vi "Weather Parse Test.vi"() -> ()   [LabVIEW 2020, in "CDM-Config.lvlib"] (continued)
008043\",\n                        \"008027\",\n                        \"008119\",\n                        \"008041\",\n                        \"008101\"\n                    ],\n                    \"UGC\": [\n                        \"COZ062\",\n                        \"COZ077\",\n                        \"COZ083\",\n                        \"COZ085\",\n                        \"COZ086\"\n                    ]\n                },\n                \"affectedZones\": [\n                    \"https://api.weather.gov/zones/forecast/COZ062\",\n                    \"https://api.weather.gov/zones/forecast/COZ077\",\n                    \"https://api.weather.gov/zones/forecast/COZ083\",\n                    \"https://api.weather.gov/zones/forecast/COZ085\",\n                    \"https://api.weather.gov/zones/forecast/COZ086\"\n                ],\n                \"references\": [\n                    {\n                        \"@id\": \"https://api.weather.gov/alerts/urn:oid:2.49.0.1.840.0.f1520a771888f2286c7e9f041b0899cca2ffbe10.006.1\",\n                        \"identifier\": \"urn:oid:2.49.0.1.840.0.f1520a771888f2286c7e9f041b0899cca2ffbe10.006.1\",\n                        \"sender\": \"w-nws.webmaster@noaa.gov\",\n                        \"sent\": \"2025-12-03T00:40:00-07:00\"\n                    },\n                    {\n                        \"@id\": \"https://api.weather.gov/alerts/urn:oid:2.49.0.1.840.0.3e97ab4a6a3c23a3a20405d82b018ef9927db31d.006.1\",\n                        \"identifier\": \"urn:oid:2.49.0.1.840.0.3e97ab4a6a3c23a3a20405d82b018ef9927db31d.006.1\",\n                        \"sender\": \"w-nws.webmaster@noaa.gov\",\n                        \"sent\": \"2025-12-03T00:46:00-07:00\"\n                    },\n                    {\n                        \"@id\": \"https://api.weather.gov/alerts/urn:oid:2.49.0.1.840.0.b7b2384d0cd65fff536137c85933eace889e9254.006.1\",\n                        \"identifier\": \"urn:oid:2.49.0.1.840.0.b7b2384d0cd65fff536137c85933eace889e9254.006.1\",\n                        \"sender\": \"w-nws.webmaster@noaa.gov\",\n                        \"sent\": \"2025-12-03T00:53:00-07:00\"\n                    },\n                    {\n                        \"@id\": \"https://api.weather.gov/alerts/urn:oid:2.49.0.1.840.0.5bb2b589973a618ffa88ed552c21d1806fce1897.006.1\",\n                        \"identifier\": \"urn:oid:2.49.0.1.840.0.5bb2b589973a618ffa88ed552c21d1806fce1897.006.1\",\n                        \"sender\": \"w-nws.webmaster@noaa.gov\",\n                        \"sent\": \"2025-12-03T02:10:00-07:00\"\n                    }\n                ],\n                \"sent\": \"2025-12-03T08:17:00-07:00\",\n                \"effective\": \"2025-12-03T08:17:00-07:00\",\n                \"onset\": \"2025-12-03T08:17:00-07:00\",\n                \"expires\": \"2025-12-03T16:30:00-07:00\",\n                \"ends\": \"2025-12-03T20:00:00-07:00\",\n                \"status\": \"Actual\",\n                \"messageType\": \"Update\",\n                \"category\": \"Met\",\n                \"severity\": \"Moderate\",\n                \"certainty\": \"Likely\",\n                \"urgency\": \"Expected\",\n                \"event\": \"Winter Weather Advisory\",\n                \"sender\": \"w-nws.webmaster@noaa.gov\",\n                \"senderName\": \"NWS Pueblo CO\",\n                \"headline\": \"Winter Weather Advisory issued December 3 at 8:17AM MST until December 3 at 8:00PM MST by NWS Pueblo CO\",\n                \"description\": \"* WHAT...Snow expected. Total snow accumulations between 2 and 8\\ninches. The heaviest snow will fall this morning into the\\nafternoon time period.\\n\\n* WHERE...Southern El Paso, Pueblo, Central Chaffee County Below\\n9000 Feet, Western/Central Fremont County Below 8500 Feet, and\\nCanon City Vicinity/Eastern Fremont County.\\n\\n* WHEN...Until 8 PM MST this evening.\\n\\n* IMPACTS...Roads, and especially bridges and overpasses, will\\nlikely become slick and hazardous. Travel could be very difficult.\\nThe hazardous conditions could impact the Wednesday evening\\ncommute.\",\n                \"instruction\": \"Slow down and use caution while traveling. The latest road\\nconditions for the state you are calling from can be obtained by\\ncalling 5 1 1.\\n\\nBe prepared for slippery roads. Slow down and use caution while\\ndriving. If you are going outside, watch your first few steps taken\\non stairs, sidewalks, and driveways. These surfaces could be icy and\\nslippery, increasing your risk of a fall and injury.\",\n                \"response\": \"Execute\",\n                \"parameters\": {\n                    \"AWIPSidentifier\": [\n                        \"WSWPUB\"\n                    ],\n                    \"WMOidentifier\": [\n                        \"WWUS45 KPUB 031517\"\n                    ],\n                    \"NWSheadline\": [\n                        \"WINTER WEATHER ADVISORY REMAINS IN EFFECT UNTIL 8 PM MST THIS EVENING\"\n                    ],\n                    \"BLOCKCHANNEL\": [\n                        \"EAS\",\n                        \"NWEM\",\n                        \"CMAS\"\n                    ],\n                    \"VTEC\": [\n                        \"/O.CON.KPUB.WW.Y.0026.000000T0000Z-251204T0300Z/\"\n                    ],\n                    \"eventEndingTime\": [\n                        \"2025-12-03T20:00:00-07:00\"\n                    ],\n                    \"expiredReferences\": [\n                        \"w-nws.webmaster@noaa.gov,urn:oid:2.49.0.1.840.0.1683fac8dbbcced155b8c3ee102b504a61d03b48.005.1,2025-12-02T21:22:00-07:00 w-nws.webmaster@noaa.gov,urn:oid:2.49.0.1.840.0.3af7c19979dcb0fd957b60f169e1bc971c265b37.007.1,2025-12-02T14:07:00-07:00 w-nws.webmaster@noaa.gov,urn:oid:2.49.0.1.840.0.3af7c19979dcb0fd957b60f169e1bc971c265b37.004.1,2025-12-02T14:07:00-07:00 w-nws.webmaster@noaa.gov,urn:oid:2.49.0.1.840.0.75fd3b8a9564f5fec4e84cc777455f52675d243c.003.1,2025-12-02T10:18:00-07:00 w-nws.webmaster@noaa.gov,urn:oid:2.49.0.1.840.0.db6c9ff9aeb621cf1cd0d104f439c64f55e7c3f7.003.1,2025-12-02T02:25:00-07:00\"\n                    ]\n                },\n                \"scope\": \"Public\",\n                \"code\": \"IPAWSv1.0\",\n                \"language\": \"en-US\",\n                \"web\": \"http://www.weather.gov\",\n                \"eventCode\": {\n                    \"SAME\": [\n                        \"NWS\"\n                    ],\n                    \"NationalWeatherService\": [\n                        \"WWY\"\n                    ]\n                }\n            }\n        },\n        {\n            \"id\": \"https://api.weather.gov/alerts/urn:oid:2.49.0.1.840.0.296069c17a90f6e5215450afb7029362483104e1.007.1\",\n            \"type\": \"Feature\",\n            \"geometry\": null,\n            \"properties\": {\n                \"@id\": \"https://api.weather.gov/alerts/urn:oid:2.49.0.1.840.0.296069c17a90f6e5215450afb7029362483104e1.007.1\",\n                \"@type\": \"wx:Alert\",\n                \"id\": \"urn:oid:2.49.0.1.840.0.296069c17a90f6e5215450afb7029362483104e1.007.1\",\n                \"areaDesc\": \"Northwestern Fremont County  Above 8500Ft\",\n                \"geocode\": {\n                    \"SAME\": [\n                        \"008043\"\n                    ],\n                    \"UGC\": [\n                        \"COZ076\"\n                    ]\n                },\n                \"affectedZones\": [\n                    \"https://api.weather.gov/zones/forecast/COZ076\"\n                ],\n                \"references\": [\n                    {\n                        \"@id\": \"https://api.weather.gov/alerts/urn:oid:2.49.0.1.840.0.f1520a771888f2286c7e9f041b0899cca2ffbe10.004.1\",\n                        \"identifier\": \"urn:oid:2.49.0.1.840.0.f1520a771888f2286c7e9f041b0899cca2ffbe10.004.1\",\n                        \"sender\": \"w-nws.webmaster@noaa.gov\",\n                        \"sent\": \"2025-12-03T00:40:00-07:00\"\n                    },\n                    {\n                        \"@id\": \"https://api.weather.gov/alerts/urn:oid:2.49.0.1.840.0.3e97ab4a6a3c23a3a20405d82b018ef9927db31d.004.1\",\n                        \"identifier\": \"urn:oid:2.49.0.1.840.0.3e97ab4a6a3c23a3a20405d82b018ef9927db31d.004.1\",\n                        \"sender\": \"w-nws.webmaster@noaa.gov\",\n                        \"sent\": \"2025-12-03T00:46:00-07:00\"\n                    },\n                    {\n                        \"@id\": \"https://api.weather.gov/alerts/urn:oid:2.49.0.1.840.0.b7b2384d0cd65fff536137c85933eace889e9254.004.1\",\n                        \"identifier\": \"urn:oid:2.49.0.1.840.0.b7b2384d0cd65fff536137c85933eace889e9254.004.1\",\n                        \"sender\": \"w-nws.webmaster@noaa.gov\",\n                        \"sent\": \"2025-12-03T00:53:00-07:00\"\n                    },\n                    {\n                        \"@id\": \"https://api.weather.gov/alerts/urn:oid:2.49.0.1.840.0.5bb2b589973a618ffa88ed552c21d1806fce1897.003.1\",\n                        \"identifier\": \"urn:oid:2.49.0.1.840.0.5bb2b589973a618ffa88ed552c21d1806fce1897.003.1\",\n                        \"sender\": \"w-nws.webmaster@noaa.gov\",\n                        \"sent\": \"2025-12-03T02:10:00-07:00\"\n                    }\n                ],\n                \"sent\": \"2025-12-03T08:17:00-07:00\",\n                \"effective\": \"2025-12-03T08:17:00-07:00\",\n                \"onset\": \"2025-12-03T08:17:00-07:00\",\n                \"expires\": \"2025-12-03T16:30:00-07:00\",\n                \"ends\": \"2025-12-03T20:00:00-07:00\",\n                \"status\": \"Actual\",\n                \"messageType\": \"Update\",\n                \"category\": \"Met\",\n                \"severity\": \"Moderate\",\n                \"certainty\": \"Likely\",\n                \"urgency\": \"Expected\",\n                \"event\": \"Winter Weather Advisory\",\n                \"sender\": \"w-nws.webmaster@noaa.gov\",\n                \"senderName\": \"NWS Pueblo CO\",\n                \"headline\": \"Winter Weather Advisory issued December 3 at 8:17AM MST until December 3 at 8:00PM MST by NWS Pueblo CO\",\n                \"description\": \"* WHAT...Snow. Additional snow accumulations between 5 to 10 inches.\\n\\n* WHERE...Northwestern Fremont County Above 8500 Feet.\\n\\n* WHEN...Until 8 PM MST this evening.\\n\\n* IMPACTS...Travel could be very difficult. The hazardous conditions\\ncould impact the Wednesday evening commute.\",\n                \"instruction\": \"Slow down and use caution while traveling. The latest road\\nconditions for the state you are calling from can be obtained by\\ncalling 5 1 1.\",\n                \"response\": \"Execute\",\n                \"parameters\": {\n                    \"AWIPSidentifier\": [\n                        \"WSWPUB\"\n                    ],\n                    \"WMOidentifier\": [\n                        \"WWUS45 KPUB 031517\"\n                    ],\n                    \"NWSheadline\": [\n                        \"WINTER WEATHER ADVISORY REMAINS IN EFFECT UNTIL 8 PM MST THIS EVENING\"\n                    ],\n                    \"BLOCKCHANNEL\": [\n                        \"EAS\",\n                        \"NWEM\",\n                        \"CMAS\"\n                    ],\n                    \"VTEC\": [\n                        \"/O.CON.KPUB.WW.Y.0026.000000T0000Z-251204T0300Z/\"\n                    ],\n                    \"eventEndingTime\": [\n                        \"2025-12-03T20:00:00-07:00\"\n                    ],\n                    \"expiredReferences\": [\n                        \"w-nws.webmaster@noaa.gov,urn:oid:2.49.0.1.840.0.1683fac8dbbcced155b8c3ee102b504a61d03b48.003.1,2025-12-02T21:22:00-07:00 w-nws.webmaster@noaa.gov,urn:oid:2.49.0.1.840.0.3af7c19979dcb0fd957b60f169e1bc971c265b37.003.1,2025-12-02T14:07:00-07:00\"\n                    ]\n                },\n                \"scope\": \"Public\",\n                \"code\": \"IPAWSv1.0\",\n                \"language\": \"en-US\",\n                \"web\": \"http://www.weather.gov\",\n                \"eventCode\": {\n                    \"SAME\": [\n                        \"NWS\"\n                    ],\n                    \"NationalWeatherService\": [\n                        \"WWY\"\n                    ]\n                }\n            }\n        },\n        {\n            \"id\": \"https://api.weather.gov/alerts/urn:oid:2.49.0.1.840.0.2ecab18b7c46d70605970fa14b41f00f24fa37fd.001.1\",\n            \"type\": \"Feature\",\n            \"geometry\": null,\n            \"properties\": {\n                \"@id\": \"https://api.weather.gov/alerts/urn:oid:2.49.0.1.840.0.2ecab18b7c46d70605970fa14b41f00f24fa37fd.001.1\",\n                \"@type\": \"wx:Alert\",\n                \"id\": \"urn:oid:2.49.0.1.840.0.2ecab18b7c46d70605970fa14b41f00f24fa37fd.001.1\",\n                \"areaDesc\": \"Coastal Gulf\",\n                \"geocode\": {\n                    \"SAME\": [\n                        \"012045\"\n                    ],\n                    \"UGC\": [\n                        \"FLZ114\"\n                    ]\n                },\n                \"affectedZones\": [\n                    \"https://api.weather.gov/zones/forecast/FLZ114\"\n                ],\n                \"references\": [],\n                \"sent\": \"2025-12-03T09:59:00-05:00\",\n                \"effective\": \"2025-12-03T09:59:00-05:00\",\n                \"onset\": \"2025-12-03T09:59:00-05:00\",\n                \"expires\": \"2025-12-03T21:00:00-05:00\",\n                \"ends\": \"2025-12-03T21:00:00-05:00\",\n                \"status\": \"Actual\",\n                \"messageType\": \"Alert\",\n                \"category\": \"Met\",\n                \"severity\": \"Moderate\",\n                \"certainty\": \"Likely\",\n                \"urgency\": \"Expected\",\n                \"event\": \"Rip Current Statement\",\n                \"sender\": \"w-nws.webmaster@noaa.gov\",\n                \"senderName\": \"NWS Tallahassee FL\",\n                \"headline\": \"Rip Current Statement issued December 3 at 9:59AM EST until December 3 at 9:00PM EST by NWS Tallahassee FL\",\n                \"description\": \"* WHAT...Dangerous rip currents.\\n\\n* WHERE...Gulf County State Park Beaches.\\n\\n* WHEN...Until 9 PM EST /8 PM CST/ this evening.\\n\\n* IMPACTS...Rip currents can sweep even the best swimmers away\\nfrom shore into deeper water.\",\n                \"instruction\": \"Swim near a lifeguard. If caught in a rip current, relax and\\nfloat. Don't swim against the current. If able, swim in a\\ndirection following the shoreline. If unable to escape, face the\\nshore and call or wave for help.\",\n                \"response\": \"Avoid\",\n                \"parameters\": {\n                    \"AWIPSidentifier\": [\n                        \"CFWTAE\"\n                    ],\n                    \"WMOidentifier\": [\n                        \"WHUS42 KTAE 031459\"\n                    ],\n                    \"NWSheadline\": [\n                        \"HIGH RIP CURRENT RISK IN EFFECT UNTIL 9 PM EST /8 PM CST/ THIS EVENING\"\n                    ],\n                    \"BLOCKCHANNEL\": [\n                        \"EAS\",\n                        \"NWEM\",\n                        \"CMAS\"\n                    ],\n                    \"VTEC\": [\n                        \"/O.NEW.KTAE.RP.S.0089.251203T1459Z-251204T0200Z/\"\n                    ],\n                    \"eventEndingTime\": [\n                        \"2025-12-03T21:00:00-05:00\"\n                    ]\n                },\n                \"scope\": \"Public\",\n                \"code\": \"IPAWSv1.0\",\n                \"language\": \"en-US\",\n                \"web\": \"http://www.weather.gov\",\n                \"eventCode\": {\n                    \"SAME\": [\n                        \"NWS\"\n                    ],\n                    \"NationalWeatherService\": [\n                        \"RPS\"\n                    ]\n                }\n            }\n        },\n        {\n            \"id\": \"https://api.weather.gov/alerts/urn:oid:2.49.0.1.840.0.2ef41cb89e608f983559be19a65d260c36845a4b.001.2\",\n            \"type\": \"Feature\",\n            \"geometry\": null,\n            \"properties\": {\n                \"@id\": \"https://api.weather.gov/alerts/urn:oid:2.49.0.1.840.0.2ef41cb89e608f983559be19a65d260c36845a4b.001.2\",\n                \"@type\": \"wx:Alert\",\n                \"id\": \"urn:oid:2.49.0.1.840.0.2ef41cb89e608f983559be19a65d260c36845a4b.001.2\",\n                \"areaDesc\": \"Coastal Waters from Eastport, ME to Schoodic Point, ME out 25 NM; Coastal Waters from Schoodic Point, ME to Stonington, ME out 25 NM\",\n                \"geocode\": {\n                    \"SAME\": [\n                        \"073050\",\n                        \"073051\"\n                    ],\n                    \"UGC\": [\n                        \"ANZ050\",\n                        \"ANZ051\"\n                    ]\n                },\n                \"affectedZones\": [\n                    \"https://api.weather.gov/zones/forecast/ANZ050\",\n                    \"https://api.weather.gov/zones/forecast/ANZ051\"\n                ],\n                \"references\": [],\n                \"sent\": \"2025-12-03T09:58:00-05:00\",\n                \"effective\": \"2025-12-03T09:58:00-05:00\",\n                \"onset\": \"2025-12-04T15:00:00-05:00\",\n                \"expires\": \"2025-12-03T18:00:00-05:00\",\n                \"ends\": \"2025-12-05T07:00:00-05:00\",\n                \"status\": \"Actual\",\n                \"messageType\": \"Alert\",\n                \"category\": \"Met\",\n                \"severity\": \"Moderate\",\n                \"certainty\": \"Likely\",\n                \"urgency\": \"Expected\",\n                \"event\": \"Gale Warning\",\n                \"sender\": \"w-nws.webmaster@noaa.gov\",\n                \"senderName\": \"NWS Caribou ME\",\n                \"headline\": \"Gale Warning issued December 3 at 9:58AM EST until December 5 at 7:00AM EST by NWS Caribou ME\",\n                \"description\": \"* WHAT...Northwest winds 30 to 40 kt and seas 7 to 10 ft\\nexpected.\\n\\n* WHERE...Coastal Waters from Eastport, ME to Schoodic Point, ME\\nout 25 NM and Coastal Waters from Schoodic Point, ME to\\nStonington, ME out 25 NM.\\n\\n* WHEN...From 3 PM Thursday to 7 AM EST Friday.\\n\\n* IMPACTS...Strong winds will cause hazardous seas which could\\ncapsize or damage vessels and reduce visibility.\",\n                \"instruction\": \"Mariners should alter plans to avoid these hazardous conditions.\\nRemain in port, seek safe harbor, alter course, and/or secure the\\nvessel for hazardous conditions.\",\n                \"response\": \"Avoid\",\n                \"parameters\": {\n                    \"AWIPSidentifier\": [\n                        \"MWWCAR\"\n                    ],\n                    \"WMOidentifier\": [\n                        \"WHUS71 KCAR 031458\"\n                    ],\n                    \"NWSheadline\": [\n                        \"GALE WARNING WILL EXPIRE AT 10 AM EST THIS MORNING... ...GALE WARNING IN EFFECT FROM 3 PM THURSDAY TO 7 AM EST FRIDAY\"\n                    ],\n                    \"BLOCKCHANNEL\": [\n                        \"EAS\",\n                        \"NWEM\",\n                        \"CMAS\"\n                    ],\n                    \"VTEC\": [\n                        \"/O.NEW.KCAR.GL.W.0035.251204T2000Z-251205T1200Z/\"\n                    ],\n                    \"eventEndingTime\": [\n                        \"2025-12-05T07:00:00-05:00\"\n                    ]\n                },\n                \"scope\": \"Public\",\n                \"code\": \"IPAWSv1.0\",\n                \"language\": \"en-US\",\n                \"web\": \"http://www.weather.gov\",\n                \"eventCode\": {\n                    \"SAME\": [\n                        \"NWS\"\n                    ],\n                    \"NationalWeatherService\": [\n                        \"GLW\"\n                    ]\n                }\n            }\n        },\n        {\n            \"id\": \"https://api.weather.gov/alerts/urn:oid:2.49.0.1.840.0.2ef41cb89e608f983559be19a65d260c36845a4b.002.2\",\n            \"type\": \"Feature\",\n            \"geometry\": null,\n            \"properties\": {\n                \"@id\": \"https://api.weather.gov/alerts/urn:oid:2.49.0.1.840.0.2ef41cb89e608f983559be19a65d260c36845a4b.002.2\",\n                \"@type\": \"wx:Alert\",\n                \"id\": \"urn:oid:2.49.0.1.840.0.2ef41cb89e608f983559be19a65d260c36845a4b.002.2\",\n                \"areaDesc\": \"Intra Coastal Waters from Schoodic Point, ME to Stonington, ME\",\n                \"geocode\": {\n                    \"SAME\": [\n                        \"073052\"\n                    ],\n                    \"UGC\": [\n                        \"ANZ052\"\n                    ]\n                },\n                \"affectedZones\": [\n                    \"https://api.weather.gov/zones/forecast/ANZ052\"\n                ],\n                \"references\": [],\n                \"sent\": \"2025-12-03T09:58:00-05:00\",\n                \"effective\": \"2025-12-03T09:58:00-05:00\",\n                \"onset\": \"2025-12-04T15:00:00-05:00\",\n                \"expires\": \"2025-12-03T18:00:00-05:00\",\n                \"ends\": \"2025-12-05T07:00:00-05:00\",\n                \"status\": \"Actual\",\n                \"messageType\": \"Alert\",\n                \"category\": \"Met\",\n                \"severity\": \"Moderate\",\n                \"certainty\": \"Likely\",\n                \"urgency\": \"Expected\",\n                \"event\": \"Gale Warning\",\n                \"sender\": \"w-nws.webmaster@noaa.gov\",\n                \"senderName\": \"NWS Caribou ME\",\n                \"headline\": \"Gale Warning issued December 3 at 9:58AM EST until December 5 at 7:00AM EST by NWS Caribou ME\",\n                \"description\": \"* WHAT...Northwest winds 25 to 35 kt with gusts up to 40 kt and\\nseas 3 to 5 ft expected.\\n\\n* WHERE...Intra Coastal Waters from Schoodic Point, ME to\\nStonington, ME.\\n\\n* WHEN...From 3 PM Thursday to 7 AM EST Friday.\\n\\n* IMPACTS...Strong winds will cause hazardous seas which could\\ncapsize or damage vessels and reduce visibility.\",\n                \"instruction\": \"Mariners should alter plans to avoid these hazardous conditions.\\nRemain in port, seek safe harbor, alter course, and/or secure the\\nvessel for hazardous conditions.\",\n                \"response\": \"Avoid\",\n                \"parameters\": {\n                    \"AWIPSidentifier\": [\n                        \"MWWCAR\"\n                    ],\n                    \"WMOidentifier\": [\n                        \"WHUS71 KCAR 031458\"\n                    ],\n                    \"NWSheadline\": [\n                        \"SMALL CRAFT ADVISORY WILL EXPIRE AT 10 AM EST THIS MORNING... ...GALE WARNING IN EFFECT FROM 3 PM THURSDAY TO 7 AM EST FRIDAY\"\n                    ],\n                    \"BLOCKCHANNEL\": [\n                        \"EAS\",\n                        \"NWEM\",\n                        \"CMAS\"\n                    ],\n                    \"VTEC\": [\n                        \"/O.NEW.KCAR.GL.W.0035.251204T2000Z-251205T1200Z/\"\n                    ],\n                    \"eventEndingTime\": [\n                        \"2025-12-05T07:00:00-05:00\"\n                    ]\n                },\n                \"scope\": \"Public\",\n                \"code\": \"IPAWSv1.0\",\n                \"language\": \"en-US\",\n                \"web\": \"http://www.weather.gov\",\n                \"eventCode\": {\n                    \"SAME\": [\n                        \"NWS\"\n                    ],\n                    \"NationalWeatherService\": [\n                        \"GLW\"\n                    ]\n                }\n            }\n        },\n        {\n            \"id\": \"https://api.weather.gov/alerts/urn:oid:2.49.0.1.840.0.58cb89d7d8c213631e5875d32db3827b35b76c1f.002.1\",\n            \"type\": \"Feature\",\n            \"geometry\": null,\n            \"properties\": {\n                \"@id\": \"https://api.weather.gov/alerts/urn:oid:2.49.0.1.840.0.58cb89d7d8c213631e5875d32db3827b35b76c1f.002.1\",\n                \"@type\": \"wx:Alert\",\n                \"id\": \"urn:oid:2.49.0.1.840.0.58cb89d7d8c213631e5875d32db3827b35b76c1f.002.1\",\n                \"areaDesc\": \"Coastal waters from Fenwick Island DE to Chincoteague VA out 20 nm; Coastal waters from Chincoteague to Parramore Island VA out 20 nm; Coastal waters from Parramore Island to Cape Charles Light VA out 20 nm; Coastal Waters from Cape Charles Light to Virginia-North Carolina border out to 20 nm; Coastal waters from NC VA border to Currituck Beach Light NC out 20 nm\",\n                \"geocode\": {\n                    \"SAME\": [\n                        \"073650\",\n                        \"073652\",\n                        \"073654\",\n                        \"073656\",\n                        \"073658\"\n                    ],\n                    \"UGC\": [\n                        \"ANZ650\",\n                        \"ANZ652\",\n                        \"ANZ654\",\n                        \"ANZ656\",\n                        \"ANZ658\"\n                    ]\n                },\n                \"affectedZones\": [\n                    \"https://api.weather.gov/zones/forecast/ANZ650\",\n                    \"https://api.weather.gov/zones/forecast/ANZ652\",\n                    \"https://api.weather.gov/zones/forecast/ANZ654\",\n                    \"https://api.weather.gov/zones/forecast/ANZ656\",\n                    \"https://api.weather.gov/zones/forecast/ANZ658\"\n                ],\n                \"references\": [\n                    {\n                        \"@id\": \"https://api.weather.gov/alerts/urn:oid:2.49.0.1.840.0.de1db5ed5596c9644ed4ea39943e7f4017835e3f.001.1\",\n                        \"identifier\": \"urn:oid:2.49.0.1.840.0.de1db5ed5596c9644ed4ea39943e7f4017835e3f.001.1\",\n                        \"sender\": \"w-nws.webmaster@noaa.gov\",\n                        \"sent\": \"2025-12-03T01:26:00-05:00\"\n                    },\n                    {\n                        \"@id\": \"https://api.weather.gov/alerts/urn:oid:2.49.0.1.840.0.7c0091d3a8b6d0ad5ccbeab61ca887dddde4ea19.002.1\",\n                        \"identifier\": \"urn:oid:2.49.0.1.840.0.7c0091d3a8b6d0ad5ccbeab61ca887dddde4ea19.002.1\",\n                        \"sender\": \"w-nws.webmaster@noaa.gov\",\n                        \"sent\": \"2025-12-03T06:40:00-05:00\"\n                    }\n                ],\n                \"sent\": \"2025-12-03T09:55:00-05:00\",\n                \"effective\": \"2025-12-03T09:55:00-05:00\",\n                \"onset\": \"2025-12-03T09:55:00-05:00\",\n                \"expires\": \"2025-12-03T12:00:00-05:00\",\n                \"ends\": \"2025-12-03T12:00:00-05:00\",\n                \"status\": \"Actual\",\n                \"messageType\": \"Update\",\n                \"category\": \"Met\",\n                \"severity\": \"Minor\",\n                \"certainty\": \"Likely\",\n                \"urgency\": \"Expected\",\n                \"event\": \"Small Craft Advisory\",\n                \"sender\": \"w-nws.webmaster@noaa.gov\",\n                \"senderName\": \"NWS Wakefield VA\",\n                \"headline\": \"Small Craft Advisory issued December 3 at 9:55AM EST until December 3 at 12:00PM EST by NWS Wakefield VA\",\n                \"description\": \"* WHAT...Northwest winds 15 kt with gusts up to 20 kt and seas 4\\nto 6 ft expected.\\n\\n* WHERE...Coastal waters from Fenwick Island DE to Chincoteague\\nVA out 20 nm, Coastal waters from Chincoteague to Parramore\\nIsland VA out 20 nm, Coastal waters from Parramore Island to\\nCape Charles Light VA out 20 nm, Coastal Waters from Cape\\nCharles Light to Virginia-North Carolina border out to 20 nm\\nand Coastal waters from NC VA border to Currituck Beach Light\\nNC out 20 nm.\\n\\n* WHEN...Until noon EST today.\\n\\n* IMPACTS...Conditions will be hazardous to small craft.\",\n                \"instruction\": \"Inexperienced mariners, especially those operating smaller\\nvessels, should avoid navigating in hazardous conditions.\",\n                \"response\": \"Avoid\",\n                \"parameters\": {\n                    \"AWIPSidentifier\": [\n                        \"MWWAKQ\"\n                    ],\n                    \"WMOidentifier\": [\n                        \"WHUS71 KAKQ 031455\"\n                    ],\n                    \"NWSheadline\": [\n                        \"SMALL CRAFT ADVISORY REMAINS IN EFFECT UNTIL NOON EST TODAY\"\n                    ],\n                    \"BLOCKCHANNEL\": [\n                        \"EAS\",\n                        \"NWEM\",\n                        \"CMAS\"\n                    ],\n                    \"VTEC\": [\n                        \"/O.CON.KAKQ.SC.Y.0132.000000T0000Z-251203T1700Z/\"\n                    ],\n                    \"eventEndingTime\": [\n                        \"2025-12-03T12:00:00-05:00\"\n                    ],\n                    \"expiredReferences\": [\n                        \"w-nws.webmaster@noaa.gov,urn:oid:2.49.0.1.840.0.bd2f073b9548e24a831e60b621ce2bfae0fe01c5.002.1,2025-12-02T18:16:00-05:00 w-nws.webmaster@noaa.gov,urn:oid:2.49.0.1.840.0.d3836c3d952d6831552aa40e60f0d224465baacf.002.1,2025-12-02T14:02:00-05:00 w-nws.webmaster@noaa.gov,urn:oid:2.49.0.1.840.0.8067bd7c44a0f9413a1f6fa02035c62b250d0bb9.001.1,2025-12-02T12:49:00-05:00 w-nws.webmaster@noaa.gov,urn:oid:2.49.0.1.840.0.ace8acc37475cfb5f1fde98a15837eaf77e14d7c.001.1,2025-12-02T10:07:00-05:00 w-nws.webmaster@noaa.gov,urn:oid:2.49.0.1.840.0.d0c36ca8333d6d10ef127a0adad97d7c3b124181.001.1,2025-12-02T04:14:00-05:00 w-nws.webmaster@noaa.gov,urn:oid:2.49.0.1.840.0.e1f75b7d7c7181ec6c439fbd046e60db0dd517a8.001.1,2025-12-01T21:07:00-05:00 w-nws.webmaster@noaa.gov,urn:oid:2.49.0.1.840.0.18a5672859a808aacd8cf4cd6d2fea72a32aeede.002.1,2025-12-01T18:42:00-05:00 w-nws.webmaster@noaa.gov,urn:oid:2.49.0.1.840.0.82e5e2cefcb3e8bb2bfb1a3d7eaa4868214af587.001.1,2025-12-01T16:06:00-05:00\"\n                    ]\n                },\n                \"scope\": \"Public\",\n                \"code\": \"IPAWSv1.0\",\n                \"language\": \"en-US\",\n                \"web\": \"http://www.weather.gov\",\n                \"eventCode\": {\n                    \"SAME\": [\n                        \"NWS\"\n                    ],\n                    \"NationalWeatherService\": [\n                        \"SCY\"\n                    ]\n                }\n            }\n        },\n        {\n            \"id\": \"https://api.weather.gov/alerts/urn:oid:2.49.0.1.840.0.999f5499b4c281d8e551528122e6e094fa9f5924.003.1\",\n            \"type\": \"Feature\",\n            \"geometry\": null,\n            \"properties\": {\n                \"@id\": \"https://api.weather.gov/alerts/urn:oid:2.49.0.1.840.0.999f5499b4c281d8e551528122e6e094fa9f5924.003.1\",\n                \"@type\": \"wx:Alert\",\n                \"id\": \"urn:oid:2.49.0.1.840.0.999f5499b4c281d8e551528122e6e094fa9f5924.003.1\",\n                \"areaDesc\": \"Detroit River Lt. to Maumee Bay OH to Reno Beach OH beyond 5NM offshoreline to US-Canadian border; Reno Beach to The Islands OH beyond 5NM off shoreline to US-Canadian border; The Islands to Vermilion OH beyond 5 nm off shoreline to US-Canadian border\",\n                \"geocode\": {\n                    \"SAME\": [\n                        \"096162\",\n                        \"096163\",\n                        \"096164\"\n                    ],\n                    \"UGC\": [\n                        \"LEZ162\",\n                        \"LEZ163\",\n                        \"LEZ164\"\n                    ]\n                },\n                \"affectedZones\": [\n                    \"https://api.weather.gov/zones/forecast/LEZ162\",\n                    \"https://api.weather.gov/zones/forecast/LEZ163\",\n                    \"https://api.weather.gov/zones/forecast/LEZ164\"\n                ],\n                \"references\": [\n                    {\n                        \"@id\": \"https://api.weather.gov/alerts/urn:oid:2.49.0.1.840.0.ddf7ebe288f35e3a560829c74d820622b2b299a4.003.1\",\n                        \"identifier\": \"urn:oid:2.49.0.1.840.0.ddf7ebe288f35e3a560829c74d820622b2b299a4.003.1\",\n                        \"sender\": \"w-nws.webmaster@noaa.gov\",\n                        \"sent\": \"2025-12-03T03:24:00-05:00\"\n                    }\n                ],\n                \"sent\": \"2025-12-03T09:42:00-05:00\",\n                \"effective\": \"2025-12-03T09:42:00-05:00\",\n                \"onset\": \"2025-12-03T10:00:00-05:00\",\n                \"expires\": \"2025-12-03T17:45:00-05:00\",\n                \"ends\": \"2025-12-03T22:00:00-05:00\",\n                \"status\": \"Actual\",\n                \"messageType\": \"Update\",\n                \"category\": \"Met\",\n                \"severity\": \"Minor\",\n                \"certainty\": \"Likely\",\n                \"urgency\": \"Expected\",\n                \"event\": \"Low Water Advisory\",\n                \"sender\": \"w-nws.webmaster@noaa.gov\",\n                \"senderName\": \"NWS Cleveland OH\",\n                \"headline\": \"Low Water Advisory issued December 3 at 9:42AM EST until December 3 at 10:00PM EST by NWS Cleveland OH\",\n                \"description\": \"* WHAT...Abnormally low water levels expected.\\n\\n* WHERE...The open waters of Lake Erie from Maumee Bay to\\nVermilion OH.\\n\\n* WHEN...From 10 AM this morning to 10 PM EST this evening.\\n\\n* IMPACTS...Below normal water levels will result in hazardous\\nnavigating conditions.\\n\\n* ADDITIONAL DETAILS...Elevated southwest winds through this\\nevening will result in water levels across the western basin\\nof Lake Erie to fall near or slightly below the critical mark\\nfor safe navigation of 5 inches below low water datum.\",\n                \"instruction\": \"Mariners should navigate shallow waters with extreme caution due\\nto below normal water levels.\",\n                \"response\": \"Avoid\",\n                \"parameters\": {\n                    \"AWIPSidentifier\": [\n                        \"MWWCLE\"\n                    ],\n                    \"WMOidentifier\": [\n                        \"WHUS71 KCLE 031442\"\n                    ],\n                    \"NWSheadline\": [\n                        \"LOW WATER ADVISORY REMAINS IN EFFECT UNTIL 10 PM EST THIS EVENING\"\n                    ],\n                    \"BLOCKCHANNEL\": [\n                        \"EAS\",\n                        \"NWEM\",\n                        \"CMAS\"\n                    ],\n                    \"VTEC\": [\n                        \"/O.CON.KCLE.LO.Y.0012.251203T1500Z-251204T0300Z/\"\n                    ],\n                    \"eventEndingTime\": [\n                        \"2025-12-03T22:00:00-05:00\"\n                    ]\n                },\n                \"scope\": \"Public\",\n                \"code\": \"IPAWSv1.0\",\n                \"language\": \"en-US\",\n                \"web\": \"http://www.weather.gov\",\n                \"eventCode\": {\n                    \"SAME\": [\n                        \"NWS\"\n                    ],\n                    \"NationalWeatherService\": [\n                        \"LOY\"\n                    ]\n                }\n            }\n        },\n        {\n            \"id\": \"https://api.weather.gov/alerts/urn:oid:2.49.0.1.840.0.999f5499b4c281d8e551528122e6e094fa9f5924.001.1\",\n            \"type\": \"Feature\",\n            \"geometry\": null,\n            \"properties\": {\n                \"@id\": \"https://api.weather.gov/alerts/urn:oid:2.49.0.1.840.0.999f5499b4c281d8e551528122e6e094fa9f5924.001.1\",\n                \"@type\": \"wx:Alert\",\n                \"id\": \"urn:oid:2.49.0.1.840.0.999f5499b4c281d8e551528122e6e094fa9f5924.001.1\",\n                \"areaDesc\": \"Maumee Bay to Reno Beach OH; Reno Beach to The Islands OH\",\n                \"geocode\": {\n                    \"SAME\": [\n                        \"096142\",\n                        \"096143\"\n                    ],\n                    \"UGC\": [\n                        \"LEZ142\",\n                        \"LEZ143\"\n                    ]\n                },\n                \"affectedZones\": [\n                    \"https://api.weather.gov/zones/forecast/LEZ142\",\n                    \"https://api.weather.gov/zones/forecast/LEZ143\"\n                ],\n                \"references\": [\n                    {\n                        \"@id\": \"https://api.weather.gov/alerts/urn:oid:2.49.0.1.840.0.ddf7ebe288f35e3a560829c74d820622b2b299a4.001.1\",\n                        \"identifier\": \"urn:oid:2.49.0.1.840.0.ddf7ebe288f35e3a560829c74d820622b2b299a4.001.1\",\n                        \"sender\": \"w-nws.webmaster@noaa.gov\",\n                        \"sent\": \"2025-12-03T03:24:00-05:00\"\n                    }\n                ],\n                \"sent\": \"2025-12-03T09:42:00-05:00\",\n                \"effective\": \"2025-12-03T09:42:00-05:00\",\n                \"onset\": \"2025-12-03T09:42:00-05:00\",\n                \"expires\": \"2025-12-03T17:45:00-05:00\",\n                \"ends\": \"2025-12-04T11:00:00-05:00\",\n                \"status\": \"Actual\",\n                \"messageType\": \"Update\",\n                \"category\": \"Met\",\n                \"severity\": \"Minor\",\n                \"certainty\": \"Likely\",\n                \"urgency\": \"Expected\",\n                \"event\": \"Small Craft Advisory\",\n                \"sender\": \"w-nws.webmaster@noaa.gov\",\n                \"senderName\": \"NWS Cleveland OH\",\n                \"headline\": \"Small Craft Advisory issued December 3 at 9:42AM EST until December 4 at 11:00AM EST by NWS Cleveland OH\",\n                \"description\": \"* WHAT...For the Small Craft Advisory, west winds to 20 knots\\nand waves 2 to 4 feet expected. For the Low Water Advisory,\\nabnormally low water levels expected.\\n\\n* WHERE...The nearshore waters of Lake Erie from Maumee Bay to\\nThe Islands OH.\\n\\n* WHEN...For the Small Craft Advisory, from 7 AM this morning to\\n11 AM EST Thursday. For the Low Water Advisory, from 10 AM\\nthis morning to 10 PM EST this evening.\\n\\n* IMPACTS...Conditions will be hazardous to small craft. Below\\nnormal water levels will result in hazardous navigating\\nconditions.\\n\\n* ADDITIONAL DETAILS...Elevated southwest winds through this\\nevening will result in water levels across the western basin\\nof Lake Erie to fall near or slightly below the critical mark\\nfor safe navigation of 5 inches below low water datum.\",\n                \"instruction\": \"Inexperienced mariners, especially those operating smaller\\nvessels, should avoid navigating in hazardous conditions.\\n\\nMariners should navigate shallow waters with extreme caution due\\nto below normal water levels.\",\n                \"response\": \"Avoid\",\n                \"parameters\": {\n                    \"AWIPSidentifier\": [\n                        \"MWWCLE\"\n                    ],\n                    \"WMOidentifier\": [\n                        \"WHUS71 KCLE 031442\"\n                    ],\n                    \"NWSheadline\": [\n                        \"SMALL CRAFT ADVISORY REMAINS IN EFFECT UNTIL 11 AM EST THURSDAY... ...LOW WATER ADVISORY REMAINS IN EFFECT UNTIL 10 PM EST THIS EVENING\"\n                    ],\n                    \"BLOCKCHANNEL\": [\n                        \"EAS\",\n                        \"NWEM\",\n                        \"CMAS\"\n                    ],\n                    \"VTEC\": [\n                        \"/O.CON.KCLE.SC.Y.0072.000000T0000Z-251204T1600Z/\"\n                    ],\n                    \"eventEndingTime\": [\n                        \"2025-12-04T11:00:00-05:00\"\n                    ],\n                    \"expiredReferences\": [\n                        \"w-nws.webmaster@noaa.gov,urn:oid:2.49.0.1.840.0.0c886383843e06dfcc6ba0a1dce77e56032b6216.001.1,2025-12-02T21:44:00-05:00\"\n                    ]\n                },\n                \"scope\": \"Public\",\n                \"code\": \"IPAWSv1.0\",\n                \"language\": \"en-US\",\n                \"web\": \"http://www.weather.gov\",\n                \"eventCode\": {\n                    \"SAME\": [\n                        \"NWS\"\n                    ],\n                    \"NationalWeatherService\": [\n                        \"SCY\"\n                    ]\n                }\n            }\n        },\n        {\n            \"id\": \"https://api.weather.gov/alerts/urn:oid:2.49.0.1.840.0.999f5499b4c281d8e551528122e6e094fa9f5924.002.2\",\n            \"type\": \"Feature\",\n            \"geometry\": null,\n            \"properties\": {\n                \"@id\": \"https://api.weather.gov/alerts/urn:oid:2.49.0.1.840.0.999f5499b4c281d8e551528122e6e094fa9f5924.002.2\",\n                \"@type\": \"wx:Alert\",\n                \"id\": \"urn:oid:2.49.0.1.840.0.999f5499b4c281d8e551528122e6e094fa9f5924.002.2\",\n                \"areaDesc\": \"The Islands to Vermilion OH\",\n                \"geocode\": {\n                    \"SAME\": [\n                        \"096144\"\n                    ],\n                    \"UGC\": [\n                        \"LEZ144\"\n                    ]\n                },\n                \"affectedZones\": [\n                    \"https://api.weather.gov/zones/forecast/LEZ144\"\n                ],\n                \"references\": [\n                    {\n                        \"@id\": \"https://api.weather.gov/alerts/urn:oid:2.49.0.1.840.0.ddf7ebe288f35e3a560829c74d820622b2b299a4.002.2\",\n                        \"identifier\": \"urn:oid:2.49.0.1.840.0.ddf7ebe288f35e3a560829c74d820622b2b299a4.002.2\",\n                        \"sender\": \"w-nws.webmaster@noaa.gov\",\n                        \"sent\": \"2025-12-03T03:24:00-05:00\"\n                    }\n                ],\n                \"sent\": \"2025-12-03T09:42:00-05:00\",\n                \"effective\": \"2025-12-03T09:42:00-05:00\",\n                \"onset\": \"2025-12-03T10:00:00-05:00\",\n                \"expires\": \"2025-12-03T17:45:00-05:00\",\n                \"ends\": \"2025-12-03T22:00:00-05:00\",\n                \"status\": \"Actual\",\n                \"messageType\": \"Update\",\n                \"category\": \"Met\",\n                \"severity\": \"Minor\",\n                \"certainty\": \"Likely\",\n                \"urgency\": \"Expected\",\n                \"event\": \"Low Water Advisory\",\n                \"sender\": \"w-nws.webmaster@noaa.gov\",\n                \"senderName\": \"NWS Cleveland OH\",\n                \"headline\": \"Low Water Advisory issued December 3 at 9:42AM EST until December 3 at 10:00PM EST by NWS Cleveland OH\",\n                \"description\": \"* WHAT...For the Small Craft Advisory, west winds to 20 knots\\nand waves 2 to 5 feet expected. For the Low Water Advisory,\\nabnormally low water levels expected.\\n\\n* WHERE...The nearshore waters of Lake Erie from The Islands to\\nVermilion OH.\\n\\n* WHEN...For the Small Craft Advisory, from 7 AM this morning to\\n7 PM EST Thursday. For the Low Water Advisory, from 10 AM this\\nmorning to 10 PM EST this evening.\\n\\n* IMPACTS...Conditions will be hazardous to small craft. Below\\nnormal water levels will result in hazardous navigating\\nconditions.\\n\\n* ADDITIONAL DETAILS...Elevated southwest winds through this\\nevening will result in water levels across the western basin\\nof Lake Erie to fall near or slightly below the critical mark\\nfor safe navigation of 5 inches below low water datum.\",\n                \"instruction\": \"Inexperienced mariners, especially those operating smaller\\nvessels, should avoid navigating in hazardous conditions.\\n\\nMariners should navigate shallow waters with extreme caution due\\nto below normal water levels.\",\n                \"response\": \"Avoid\",\n                \"parameters\": {\n                    \"AWIPSidentifier\": [\n                        \"MWWCLE\"\n                    ],\n                    \"WMOidentifier\": [\n                        \"WHUS71 KCLE 031442\"\n                    ],\n                    \"NWSheadline\": [\n                        \"SMALL CRAFT ADVISORY REMAINS IN EFFECT UNTIL 7 PM EST THURSDAY... ...LOW WATER ADVISORY REMAINS IN EFFECT UNTIL 10 PM EST THIS EVENING\"\n                    ],\n                    \"BLOCKCHANNEL\": [\n                        \"EAS\",\n                        \"NWEM\",\n                        \"CMAS\"\n                    ],\n                    \"VTEC\": [\n                        \"/O.CON.KCLE.LO.Y.0012.251203T1500Z-251204T0300Z/\"\n                    ],\n                    \"eventEndingTime\": [\n                        \"2025-12-03T22:00:00-05:00\"\n                    ]\n                },\n                \"scope\": \"Public\",\n                \"code\": \"IPAWSv1.0\",\n                \"language\": \"en-US\",\n                \"web\": \"http://www.weather.gov\",\n                \"eventCode\": {\n                    \"SAME\": [\n                        \"NWS\"\n                    ],\n                    \"NationalWeatherService\": [\n                        \"LOY\"\n                    ]\n                }\n            }\n        },\n        {\n            \"id\": \"https://api.weather.gov/alerts/urn:oid:2.49.0.1.840.0.999f5499b4c281d8e551528122e6e094fa9f5924.001.2\",\n            \"type\": \"Feature\",\n            \"geometry\": null,\n            \"properties\": {\n                \"@id\": \"https://api.weather.gov/alerts/urn:oid:2.49.0.1.840.0.999f5499b4c281d8e551528122e6e094fa9f5924.001.2\",\n                \"@type\": \"wx:Alert\",\n                \"id\": \"urn:oid:2.49.0.1.840.0.999f5499b4c281d8e551528122e6e094fa9f5924.001.2\",\n                \"areaDesc\": \"Maumee Bay to Reno Beach OH; Reno Beach to The Islands OH\",\n                \"geocode\": {\n                    \"SAME\": [\n                        \"096142\",\n                        \"096143\"\n                    ],\n                    \"UGC\": [\n                        \"LEZ142\",\n                        \"LEZ143\"\n                    ]\n                },\n                \"affectedZones\": [\n                    \"https://api.weather.gov/zones/forecast/LEZ142\",\n                    \"https://api.weather.gov/zones/forecast/LEZ143\"\n                ],\n                \"references\": [\n                    {\n                        \"@id\": \"https://api.weather.gov/alerts/urn:oid:2.49.0.1.840.0.ddf7ebe288f35e3a560829c74d820622b2b299a4.001.2\",\n                        \"identifier\": \"urn:oid:2.49.0.1.840.0.ddf7ebe288f35e3a560829c74d820622b2b299a4.001.2\",\n                        \"sender\": \"w-nws.webmaster@noaa.gov\",\n                        \"sent\": \"2025-12-03T03:24:00-05:00\"\n                    }\n                ],\n                \"sent\": \"2025-12-03T09:42:00-05:00\",\n                \"effective\": \"2025-12-03T09:42:00-05:00\",\n                \"onset\": \"2025-12-03T10:00:00-05:00\",\n                \"expires\": \"2025-12-03T17:45:00-05:00\",\n                \"ends\": \"2025-12-03T22:00:00-05:00\",\n                \"status\": \"Actual\",\n                \"messageType\": \"Update\",\n                \"category\": \"Met\",\n                \"severity\": \"Minor\",\n                \"certainty\": \"Likely\",\n                \"urgency\": \"Expected\",\n                \"event\": \"Low Water Advisory\",\n                \"sender\": \"w-nws.webmaster@noaa.gov\",\n                \"senderName\": \"NWS Cleveland OH\",\n                \"headline\": \"Low Water Advisory issued December 3 at 9:42AM EST until December 3 at 10:00PM EST by NWS Cleveland OH\",\n                \"description\": \"* WHAT...For the Small Craft Advisory, west winds to 20 knots\\nand waves 2 to 4 feet expected. For the Low Water Advisory,\\nabnormally low water levels expected.\\n\\n* WHERE...The nearshore waters of Lake Erie from Maumee Bay to\\nThe Islands OH.\\n\\n* WHEN...For the Small Craft Advisory, from 7 AM this morning to\\n11 AM EST Thursday. For the Low Water Advisory, from 10 AM\\nthis morning to 10 PM EST this evening.\\n\\n* IMPACTS...Conditions will be hazardous to small craft. Below\\nnormal water levels will result in hazardous navigating\\nconditions.\\n\\n* ADDITIONAL DETAILS...Elevated southwest winds through this\\nevening will result in water levels across the western basin\\nof Lake Erie to fall near or slightly below the critical mark\\nfor safe navigation of 5 inches below low water datum.\",\n                \"instruction\": \"Inexperienced mariners, especially those operating smaller\\nvessels, should avoid navigating in hazardous conditions.\\n\\nMariners should navigate shallow waters with extreme caution due\\nto below normal water levels.\",\n                \"response\": \"Avoid\",\n                \"parameters\": {\n                    \"AWIPSidentifier\": [\n                        \"MWWCLE\"\n                    ],\n                    \"WMOidentifier\": [\n                        \"WHUS71 KCLE 031442\"\n                    ],\n                    \"NWSheadline\": [\n                        \"SMALL CRAFT ADVISORY REMAINS IN EFFECT UNTIL 11 AM EST THURSDAY... ...LOW WATER ADVISORY REMAINS IN EFFECT UNTIL 10 PM EST THIS EVENING\"\n                    ],\n                    \"BLOCKCHANNEL\": [\n                        \"EAS\",\n                        \"NWEM\",\n                        \"CMAS\"\n                    ],\n                    \"VTEC\": [\n                        \"/O.CON.KCLE.LO.Y.0012.251203T1500Z-251204T0300Z/\"\n                    ],\n                    \"eventEndingTime\": [\n                        \"2025-12-03T22:00:00-05:00\"\n                    ]\n                },\n                \"scope\": \"Public\",\n                \"code\": \"IPAWSv1.0\",\n                \"language\": \"en-US\",\n                \"web\": \"http://www.weather.gov\",\n                \"eventCode\": {\n                    \"SAME\": [\n                        \"NWS\"\n                    ],\n                    \"NationalWeatherService\": [\n                        \"LOY\"\n                    ]\n                }\n            }\n        },\n        {\n            \"id\": \"https://api.weather.gov/alerts/urn:oid:2.49.0.1.840.0.999f5499b4c281d8e551528122e6e094fa9f5924.004.1\",\n            \"type\": \"Feature\",\n            \"geometry\": null,\n            \"properties\": {\n                \"@id\": \"https://api.weather.gov/alerts/urn:oid:2.49.0.1.840.0.999f5499b4c281d8e551528122e6e094fa9f5924.004.1\",\n                \"@type\": \"wx:Alert\",\n                \"id\": \"urn:oid:2.49.0.1.840.0.999f5499b4c281d8e551528122e6e094fa9f5924.004.1\",\n                \"areaDesc\": \"Vermilion to Avon Point OH; Avon Point to Willowick OH; Willowick to Geneva-on-the Lake OH; Geneva-on-the-Lake to Conneaut OH; Conneaut OH to Ripley NY\",\n                \"geocode\": {\n                    \"SAME\": [\n                        \"096145\",\n                        \"096146\",\n                        \"096147\",\n                        \"096148\",\n                        \"096149\"\n                    ],\n                    \"UGC\": [\n                        \"LEZ145\",\n                        \"LEZ146\",\n                        \"LEZ147\",\n                        \"LEZ148\",\n                        \"LEZ149\"\n                    ]\n                },\n                \"affectedZones\": [\n                    \"https://api.weather.gov/zones/forecast/LEZ145\",\n                    \"https://api.weather.gov/zones/forecast/LEZ146\",\n                    \"https://api.weather.gov/zones/forecast/LEZ147\",\n                    \"https://api.weather.gov/zones/forecast/LEZ148\",\n                    \"https://api.weather.gov/zones/forecast/LEZ149\"\n                ],\n                \"references\": [\n                    {\n                        \"@id\": \"https://api.weather.gov/alerts/urn:oid:2.49.0.1.840.0.ddf7ebe288f35e3a560829c74d820622b2b299a4.004.1\",\n                        \"identifier\": \"urn:oid:2.49.0.1.840.0.ddf7ebe288f35e3a560829c74d820622b2b299a4.004.1\",\n                        \"sender\": \"w-nws.webmaster@noaa.gov\",\n                        \"sent\": \"2025-12-03T03:24:00-05:00\"\n                    },\n                    {\n                        \"@id\": \"https://api.weather.gov/alerts/urn:oid:2.49.0.1.840.0.ddf7ebe288f35e3a560829c74d820622b2b299a4.005.1\",\n                        \"identifier\": \"urn:oid:2.49.0.1.840.0.ddf7ebe288f35e3a560829c74d820622b2b299a4.005.1\",\n                        \"sender\": \"w-nws.webmaster@noaa.gov\",\n                        \"sent\": \"2025-12-03T03:24:00-05:00\"\n                    }\n                ],\n                \"sent\": \"2025-12-03T09:42:00-05:00\",\n                \"effective\": \"2025-12-03T09:42:00-05:00\",\n                \"onset\": \"2025-12-03T09:42:00-05:00\",\n                \"expires\": \"2025-12-03T17:45:00-05:00\",\n                \"ends\": \"2025-12-04T19:00:00-05:00\",\n                \"status\": \"Actual\",\n                \"messageType\": \"Update\",\n                \"category\": \"Met\",\n                \"severity\": \"Minor\",\n                \"certainty\": \"Likely\",\n                \"urgency\": \"Expected\",\n                \"event\": \"Small Craft Advisory\",\n                \"sender\": \"w-nws.webmaster@noaa.gov\",\n                \"senderName\": \"NWS Cleveland OH\",\n                \"headline\": \"Small Craft Advisory issued December 3 at 9:42AM EST until December 4 at 7:00PM EST by NWS Cleveland OH\",\n                \"description\": \"* WHAT...West winds 15 to 25 knots and waves 4 to 7 feet\\nexpected.\\n\\n* WHERE...The nearshore waters of Lake Erie from Vermilion to\\nConneaut OH.\\n\\n* WHEN...From 7 AM this morning to 7 PM EST Thursday.\\n\\n* IMPACTS...Conditions will be hazardous to small craft.\",\n                \"instruction\": \"Inexperienced mariners, especially those operating smaller\\nvessels, should avoid navigating in hazardous conditions.\",\n                \"response\": \"Avoid\",\n                \"parameters\": {\n                    \"AWIPSidentifier\": [\n                        \"MWWCLE\"\n                    ],\n                    \"WMOidentifier\": [\n                        \"WHUS71 KCLE 031442\"\n                    ],\n                    \"NWSheadline\": [\n                        \"SMALL CRAFT ADVISORY REMAINS IN EFFECT UNTIL 7 PM EST THURSDAY\"\n                    ],\n                    \"BLOCKCHANNEL\": [\n                        \"EAS\",\n                        \"NWEM\",\n                        \"CMAS\"\n                    ],\n                    \"VTEC\": [\n                        \"/O.CON.KCLE.SC.Y.0072.000000T0000Z-251205T0000Z/\"\n                    ],\n                    \"eventEndingTime\": [\n                        \"2025-12-04T19:00:00-05:00\"\n                    ],\n                    \"expiredReferences\": [\n                        \"w-nws.webmaster@noaa.gov,urn:oid:2.49.0.1.840.0.0c886383843e06dfcc6ba0a1dce77e56032b6216.003.1,2025-12-02T21:44:00-05:00 w-nws.webmaster@noaa.gov,urn:oid:2.49.0.1.840.0.0c886383843e06dfcc6ba0a1dce77e56032b6216.002.1,2025-12-02T21:44:00-05:00\"\n                    ]\n                },\n                \"scope\": \"Public\",\n                \"code\": \"IPAWSv1.0\",\n                \"language\": \"en-US\",\n                \"web\": \"http://www.weather.gov\",\n                \"eventCode\": {\n                    \"SAME\": [\n                        \"NWS\"\n                    ],\n                    \"NationalWeatherService\": [\n                        \"SCY\"\n                    ]\n                }\n            }\n        },\n        {\n            \"id\": \"https://api.weather.gov/alerts/urn:oid:2.49.0.1.840.0.999f5499b4c281d8e551528122e6e094fa9f5924.002.1\",\n            \"type\": \"Feature\",\n            \"geometry\": null,\n            \"properties\": {\n                \"@id\": \"https://api.weather.gov/alerts/urn:oid:2.49.0.1.840.0.999f5499b4c281d8e551528122e6e094fa9f5924.002.1\",\n                \"@type\": \"wx:Alert\",\n                \"id\": \"urn:oid:2.49.0.1.840.0.999f5499b4c281d8e551528122e6e094fa9f5924.002.1\",\n                \"areaDesc\": \"The Islands to Vermilion OH\",\n                \"geocode\": {\n                    \"SAME\": [\n                        \"096144\"\n                    ],\n                    \"UGC\": [\n                        \"LEZ144\"\n                    ]\n                },\n                \"affectedZones\": [\n                    \"https://api.weather.gov/zones/forecast/LEZ144\"\n                ],\n                \"references\": [\n                    {\n                        \"@id\": \"https://api.weather.gov/alerts/urn:oid:2.49.0.1.840.0.ddf7ebe288f35e3a560829c74d820622b2b299a4.002.1\",\n                        \"identifier\": \"urn:oid:2.49.0.1.840.0.ddf7ebe288f35e3a560829c74d820622b2b299a4.002.1\",\n                        \"sender\": \"w-nws.webmaster@noaa.gov\",\n                        \"sent\": \"2025-12-03T03:24:00-05:00\"\n                    }\n                ],\n                \"sent\": \"2025-12-03T09:42:00-05:00\",\n                \"effective\": \"2025-12-03T09:42:00-05:00\",\n                \"onset\": \"2025-12-03T09:42:00-05:00\",\n                \"expires\": \"2025-12-03T17:45:00-05:00\",\n                \"ends\": \"2025-12-04T19:00:00-05:00\",\n                \"status\": \"Actual\",\n                \"messageType\": \"Update\",\n                \"category\": \"Met\",\n                \"severity\": \"Minor\",\n                \"certainty\": \"Likely\",\n                \"urgency\": \"Expected\",\n                \"event\": \"Small Craft Advisory\",\n                \"sender\": \"w-nws.webmaster@noaa.gov\",\n                \"senderName\": \"NWS Cleveland OH\",\n                \"headline\": \"Small Craft Advisory issued December 3 at 9:42AM EST until December 4 at 7:00PM EST by NWS Cleveland OH\",\n                \"description\": \"* WHAT...For the Small Craft Advisory, west winds to 20 knots\\nand waves 2 to 5 feet expected. For the Low Water Advisory,\\nabnormally low water levels expected.\\n\\n* WHERE...The nearshore waters of Lake Erie from The Islands to\\nVermilion OH.\\n\\n* WHEN...For the Small Craft Advisory, from 7 AM this morning to\\n7 PM EST Thursday. For the Low Water Advisory, from 10 AM this\\nmorning to 10 PM EST this evening.\\n\\n* IMPACTS...Conditions will be hazardous to small craft. Below\\nnormal water levels will result in hazardous navigating\\nconditions.\\n\\n* ADDITIONAL DETAILS...Elevated southwest winds through this\\nevening will result in water levels across the western basin\\nof Lake Erie to fall near or slightly below the critical mark\\nfor safe navigation of 5 inches below low water datum.\",\n                \"instruction\": \"Inexperienced mariners, especially those operating smaller\\nvessels, should avoid navigating in hazardous conditions.\\n\\nMariners should navigate shallow waters with extreme caution due\\nto below normal water levels.\",\n                \"response\": 
